vi "REV Get Sensor Values.vi"() -> ()   [LabVIEW 2020]
uses:
  <vilib>/Rock Robotics/SystemInterfaces/DIO/FPGA_DIOPWMChannel.ctl
  <vilib>/Rock Robotics/WPI/PWM/WPI_PWMDeadband.ctl
  <vilib>/Rock Robotics/WPI/MotorControl/WPI_MotorControlType.ctl
  <vilib>/Rock Robotics/SystemInterfaces/DIO/FPGA_DIOChannel.ctl
  <vilib>/Rock Robotics/WPI/MotorControl/WPI_MotorControlDeviceRef.ctl
  Type Definitions/Hardware/4 Motor Sets/(Falcon 500) 4 Motor Set.ctl
  Type Definitions/Hardware/Swerve Drives/(Falcon-Falcon-CANCoder-Pigeon2) Swerve.ctl
panel:
  out "Steer Angles (rotations)":T1
  out "Drive Velocities (RPM)":T1
  out "Steer Angles (degrees)":T2
  out "Drive Velocities (ft/s)":T2
  in  "REV Motors":T3
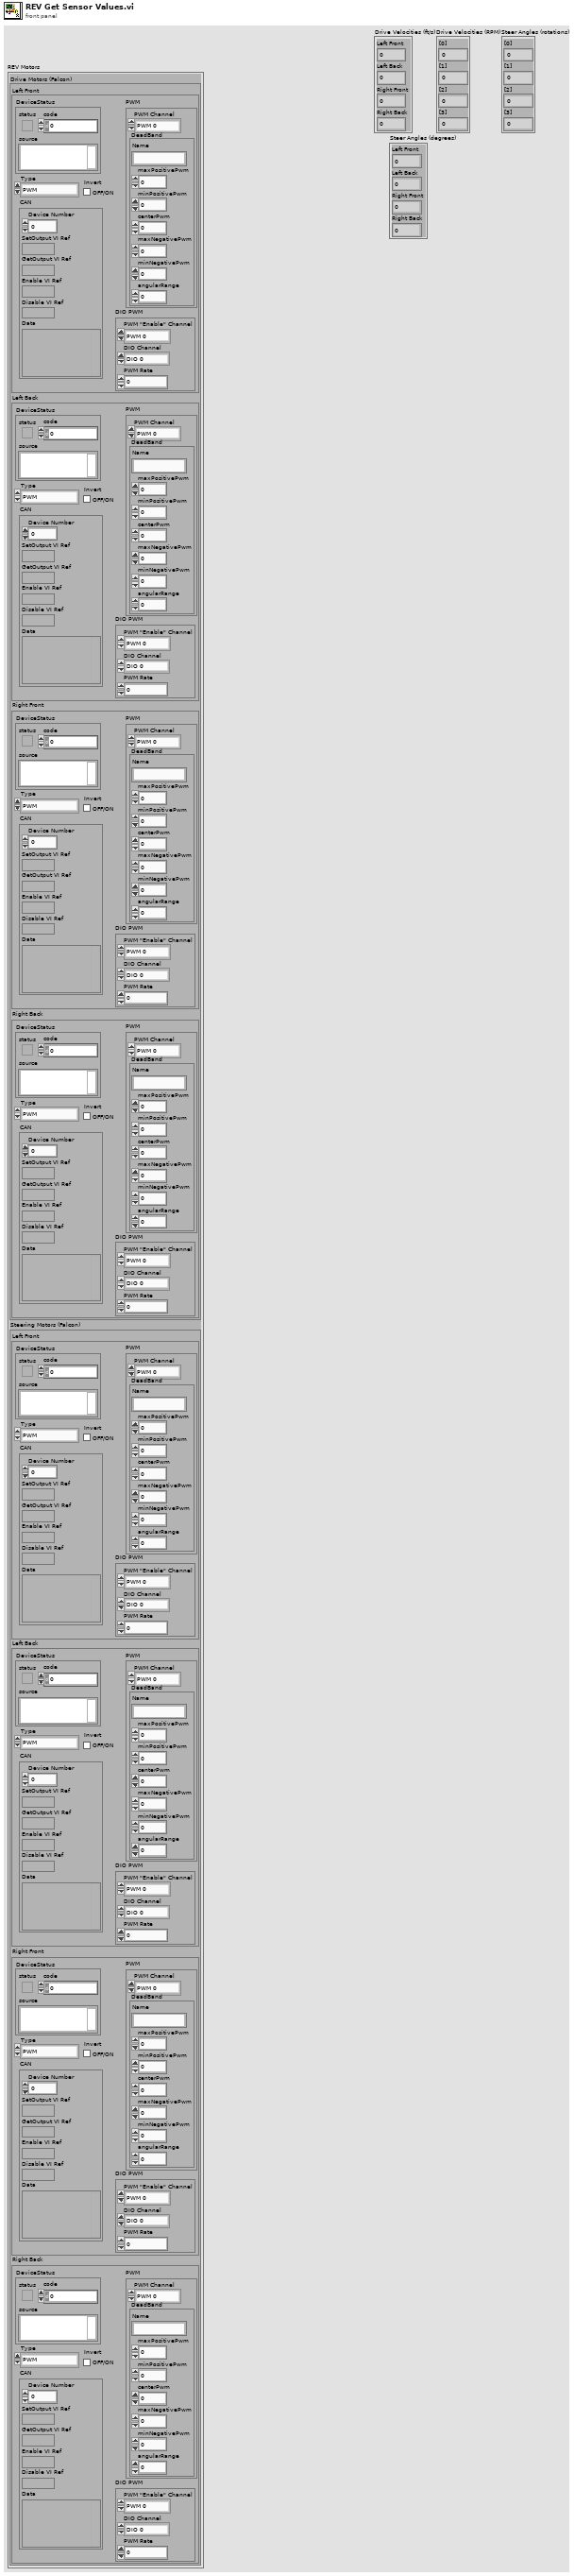
[diagram p1: front panel]
types:
  T1 = cluster{"[0]":dbl, "[1]":dbl, "[2]":dbl, "[3]":dbl}
  T2 = cluster{"Left Front":dbl, "Left Back":dbl, "Right Front":dbl, "Right Back":dbl}
  T3 = typedef "(Falcon-Falcon-CANCoder-Pigeon2) Swerve.ctl" = cluster{"Drive Motors (Falcon)":T4, "Steering Motors (Falcon)":T4}
  T4 = typedef "(Falcon 500) 4 Motor Set.ctl" = cluster{"Left Front":T5, "Left Back":T5, "Right Front":T5, "Right Back":T5}
  T5 = typedef "WPI_MotorControlDeviceRef.ctl" = cluster{"DeviceStatus":errorcluster, "Type":T6, "PWM":cluster{"PWM Channel":T7, "DeadBand":T8}, "CAN":cluster{"Device Number":u8, "SetOutput VI Ref":variant, "GetOutput VI Ref":variant, "Enable VI Ref":variant, "Disable VI Ref":variant, "Data":variant}, "Invert":bool, "DIO PWM":cluster{"PWM \"Enable\" Channel":T7, "DIOChannel":T9, "PWM Rate":dbl}}
  T6 = typedef "WPI_MotorControlType.ctl" = enum16{"PWM", "CAN", "DIO PWM"}
  T7 = typedef "FPGA_DIOPWMChannel.ctl" = enum8{"PWM 0", "PWM 1", "PWM 2", "PWM 3", "PWM 4", "PWM 5", "PWM 6", "PWM 7", "PWM 8", "PWM 9", "PWM MXP 0", "PWM MXP 1", "PWM MXP 2", "PWM MXP 3", "PWM MXP 4", "PWM MXP 5", "PWM MXP 6", "PWM MXP 7", "PWM MXP 8", "PWM MXP 9", "Invalid"}
  T8 = typedef "WPI_PWMDeadband.ctl" = cluster{"Name":string, "maxPositivePwm":i32, "minPositivePwm":i32, "centerPwm":i32, "maxNegativePwm":i32, "minNegativePwm":i32, "angularRange":u16}
  T9 = typedef "FPGA_DIOChannel.ctl" = enum8{"DIO 0", "DIO 1", "DIO 2", "DIO 3", "DIO 4", "DIO 5", "DIO 6", "DIO 7", "DIO 8", "DIO 9", "DIO MXP 0", "DIO MXP 1", "DIO MXP 2", "DIO MXP 3", "DIO MXP 4", "DIO MXP 5", "DIO MXP 6", "DIO MXP 7", "DIO MXP 8", "DIO MXP 9", "DIO MXP 10", "DIO MXP 11", "DIO MXP 12", "DIO MXP 13", "DIO MXP 14", "DIO MXP 15", "SPI Port CS1", "SPI Port CS2", "SPI Port CS3", "SPI Port MISO", "SPI Port MOSI", "Invalid"}
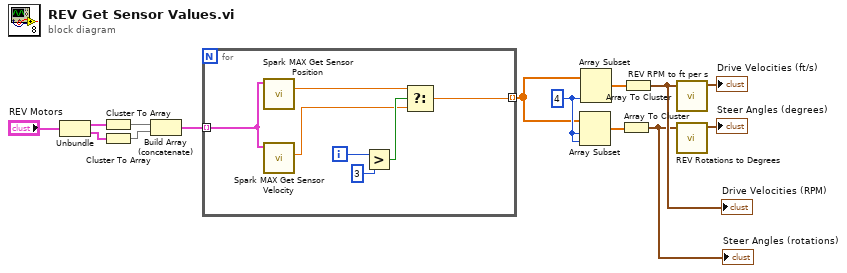
[diagram p0: block diagram]
diagram:
  w6 = 4 ("length")
  n1 = Unbundle("REV Motors") -> ("Drive Motors (Falcon)"=w13:T4, "Steering Motors (Falcon)"=w12:T4)
  n2 = Cluster To Array(cluster=w13) -> (array=w11:T5[])
  n3 = Cluster To Array(cluster=w12) -> (array=w10:T5[])
  n4 = Build Array (concatenate)(w11, w10) -> (w9:T5[])
  n5 = for {
    tunnel: w9 -> [w21] mode=indexing
    tunnel: [w15] -> w5 mode=indexing
    i -> [w17]
    n6 = call <vilib>:"Spark MAX Get Sensor Position.vi"("MotorControlDevRef in"=w21) -> ("Sensor Position"=w18:dbl)  [unwired: 7 in, 3 out]
    n7 = call <vilib>:"Spark MAX Get Sensor Velocity.vi"("MotorControlDevRef in"=w21) -> ("Sensor Velocity"=w16:dbl)  [unwired: 7 in, 3 out]
    n8 = Greater?(x=w17, y=3) -> (0:w19:bool)
    n9 = Select(t=w18, s=w19, f=w16) -> (s? t:f=w15:dbl)
  }
  n10 = Array Subset(array=w5, index=w6, length=w6) -> (w8:dbl[])
  n11 = Array Subset(array=w5, length=w6) -> (w7:dbl[])  [unwired: 1 in]
  n12 = Array To Cluster(array=w8) -> (cluster=w1:T1)
  "Steer Angles (rotations)" <- w1
  n13 = Array To Cluster(array=w7) -> (cluster=w2:T1)
  "Drive Velocities (RPM)" <- w2
  n14 = call "REV RPM to ft per s.vi"("Drive Velocities (RPM)"=w2) -> ("Drive Velocities (ft/s)"=→"Drive Velocities (ft/s)":T2)  [unwired: 10 in]
  n15 = call "REV Rotations to Degrees.vi"("Steer Angles (rotations)"=w1) -> ("Steer Angles (degrees)"=→"Steer Angles (degrees)":T2)  [unwired: 10 in]
